vi "Focus Index by Grids.vi"(0 "Input array":dbl[][][][](array[numeric]), 1 "Primary X index":u8=1, 2 "Smoothing radius 1":u16=1, 3 "Smoothing radius 2":u16=4, 5 "X grids":u8=1, 6 "Pre-bin 2":bool=TRUE, 7 "Y grids":u8=1, 9 "X length":u32, 11 "Y length":u32, 12 "Primary Y index":u8=1) -> (4 "Focus index array":sgl[][](array[numeric]), 8 "Primary FI":sgl, 13 "Primary eval area mean":sgl format="%0.2f", 14 "Primary eval area std":sgl format="%0.2f", 15 "Primary eval area":dbl[][](graph))   [LabVIEW 2018]
uses:
  <vilib>/Analysis/NI_AALBase.lvlib
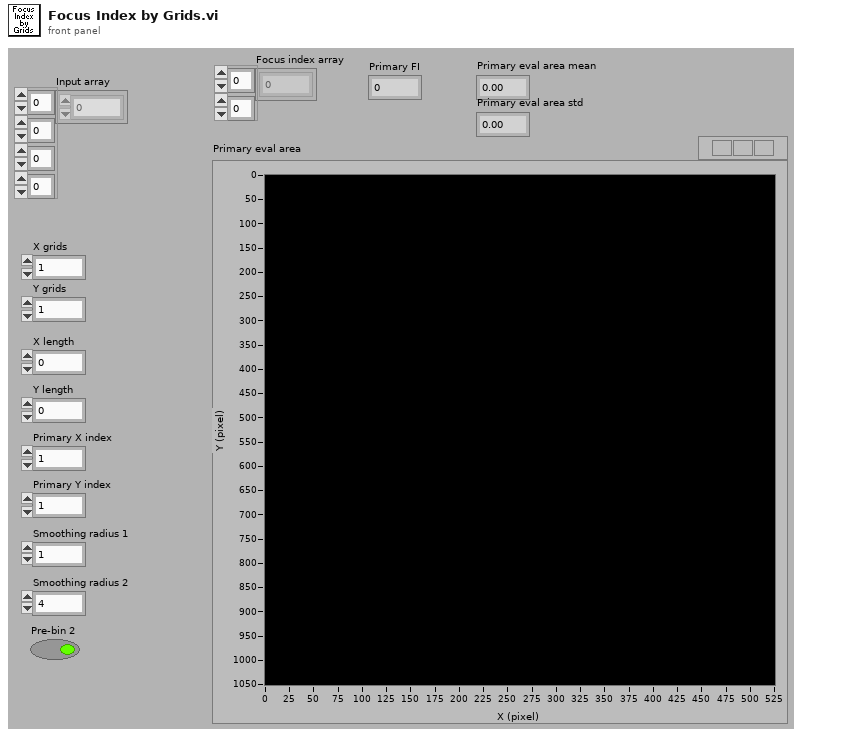
[diagram p1: front panel]
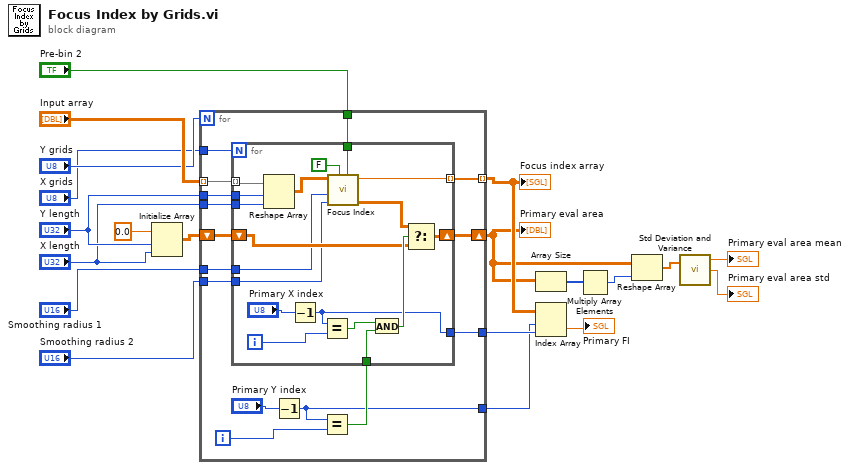
[diagram p0: block diagram]
diagram:
  n1 = Initialize Array(0.0 ("element"), "Y length", "X length") -> (w19:dbl[][])
  n2 = for {
    N: "Y grids" -> [_]
    tunnel: "Input array" -> [w35] mode=indexing
    tunnel: [w34] -> w14 mode=indexing
    tunnel: "X length" -> [w33]
    tunnel: "Y length" -> [w32]
    shift-right: [w29] -> w8
    shift-left: w19 -> [w28]
    tunnel: "Smoothing radius 1" -> [w27]
    tunnel: "Smoothing radius 2" -> [w26]
    tunnel: [w25] -> w13
    tunnel: [w23] -> w12
    tunnel: "Pre-bin 2" -> [w22]
    tunnel: "X grids" -> [w21]
    i -> [w31]
    n3 = Decrement(x="Primary Y index") -> (x-1=w23:u8)
    n4 = Equal?(x=w23, y=w31) -> (x = y?=w30:bool)
    n5 = for {
      N: w21 -> [_]
      tunnel: w35 -> [w49] mode=indexing
      tunnel: [w53] -> w34 mode=indexing
      tunnel: w33 -> [w52]
      tunnel: w32 -> [w51]
      tunnel: w30 -> [w45]
      shift-right: [w42] -> w29
      shift-left: w28 -> [w41]
      tunnel: w27 -> [w40]
      tunnel: w26 -> [w39]
      tunnel: [w37] -> w25
      tunnel: w22 -> [w36]
      i -> [w47]
      n6 = Reshape Array(w49, w51, w52) -> (w48:dbl[][])
      n7 = Decrement(x="Primary X index") -> (x-1=w37:u8)
      n8 = Equal?(x=w37, y=w47) -> (x = y?=w46:bool)
      n9 = call "Focus Index.vi"("Pre-bin 2"=w36, "Limit area"=FALSE, "Smoothing radius 2"=w39, "Smoothing radius 1"=w40, "Input"=w48) -> ("Eval area"=w43:dbl[][], "Focus index"=w53:sgl)  [unwired: 5 in]
      n10 = And(x=w46, y=w45) -> (x .and. y?=w44:bool)
      n11 = Select(t=w43, s=w44, f=w41) -> (s? t:f=w42:dbl[][])
    }
  }
  "Focus index array" <- w14
  "Primary eval area" <- w8
  n12 = Array Size(array=w8) -> (size(s)=w10:i32[])
  n13 = Index Array(array=w14, index (row)=w12, index (col)=w13) -> (element=→"Primary FI":sgl)
  n14 = Multiply Array Elements(1:w10) -> (0:w9:i32)
  n15 = Reshape Array(w8, w9) -> (w7:dbl[])
  n16 = call <vilib>:"Std Deviation and Variance.vi"("X"=w7) -> ("mean"=→"Primary eval area mean":dbl, "standard deviation"=→"Primary eval area std":dbl)  [unwired: 1 in, 1 out]
